vi "Get Container ACL.vi"(8 "error in (no error)":errorcluster, 10 "Container":string, 11 "Azure Session in":refnum<class "Session.lvclass">) -> (0 "error out":errorcluster, 2 "ACL":T1[](array[typedef]), 3 "Azure Session out":refnum<class "Session.lvclass">)   [LabVIEW 2015, in "NI_Azure_Blob.lvlib"]
doc: "Gets the public access policy and any stored access policies for the container."
uses:
  NI_Azure_Blob.lvlib
  Core/Session/Session.lvclass
  Signed Identifier.ctl
  Access Policy.ctl
  Core/Name Value Pair.ctl
  Core/Session/Session.lvclass/Session.ctl
  Core/Session/Write Request Parameters.vi
  Core/Session/Write HTTP Verb.vi
  Core/Session/Write URL Suffix.vi
  Core/NI_Azure_Core.lvlib
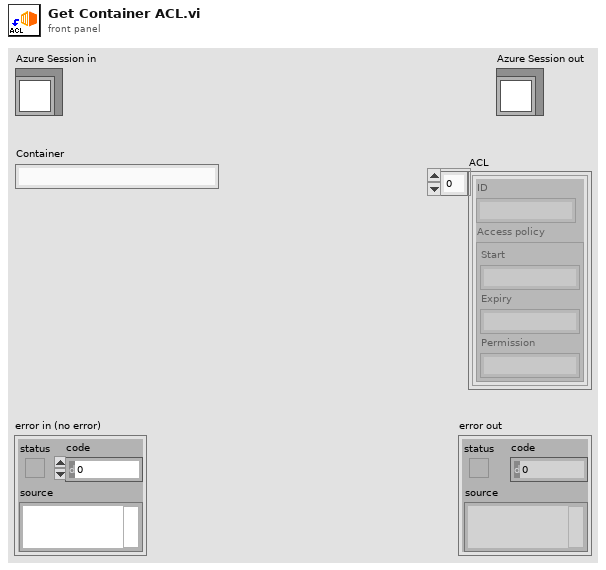
[diagram p1: front panel]
types:
  T1 = typedef "NI_Azure_Blob.lvlib/Signed Identifier.ctl" = cluster{"ID":string, "Access policy":T2}
  T2 = typedef "NI_Azure_Blob.lvlib/Access Policy.ctl" = cluster{"Start":string, "Expiry":string, "Permission":string}
  T3 = typedef "NI_Azure_Core.lvlib/Name Value Pair.ctl" = cluster{"name":string, "value":string}
  T4 = typedef "NI_Azure_Core.lvlib/Response.ctl" = cluster{"Headers":string, "Body":string}
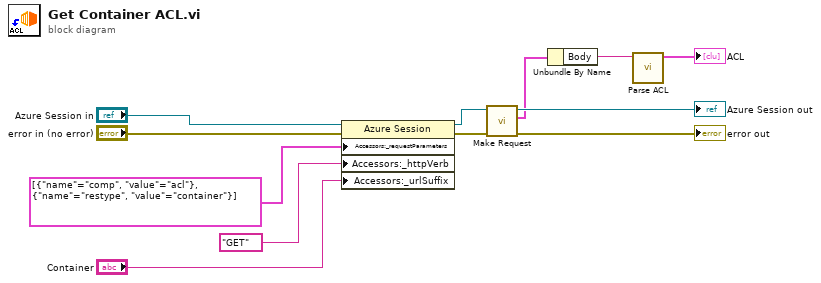
[diagram p0: block diagram]
diagram:
  n1 = property class="Azure Session"(reference="Azure Session in", error in="error in (no error)", "Accessors:_requestParameters"=T3[] [{"name"="comp", "value"="acl"}, {"name"="restype", "value"="container"}] ("request parameters"), "Accessors:_httpVerb"="GET" ("HTTP-Verb"), "Accessors:_urlSuffix"="Container") -> (reference out=w4:refnum<class "Session.lvclass">, error out=w6:errorcluster)
  n2 = call "Make Request.vi"("error in (no error)"=w6, "Session in"=w4) -> ("error out"=→"error out":errorcluster, "Response"=w7:T4, "Session out"=→"Azure Session out":refnum<class "Session.lvclass">)  [unwired: 7 in]
  n3 = Unbundle By Name(w7) -> ("Body"=w8:string)
  n4 = call "Parse ACL.vi"("String"=w8) -> ("Signed identifiers"=→"ACL":T1[])  [unwired: 10 in]
